vi "GetAlarms.vi"(0 "Valve_2DO_2DI in":refnum<class "Valve_2DO_2DI.lvclass">, 11 "error in (no error)":errorcluster) -> (4 "Valve_2DO_2DI out":refnum<class "Valve_2DO_2DI.lvclass">, 6 "Alarm":bool, 8 "Warning":bool, 15 "error out":errorcluster)   [LabVIEW 2019, in "Valve_2DO_2DI.lvclass"]
uses:
  Valve_2DO_2DI.lvclass
  Valve_2DO_2DI.lvclass/Valve_2DO_2DI.ctl
  DA_class/DA.lvclass
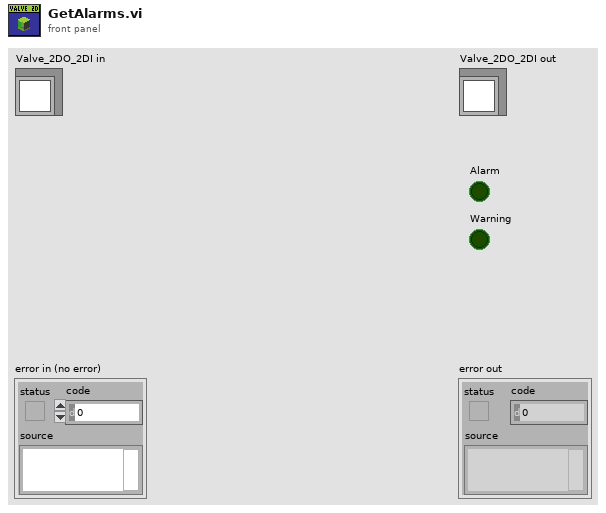
[diagram p1: front panel]
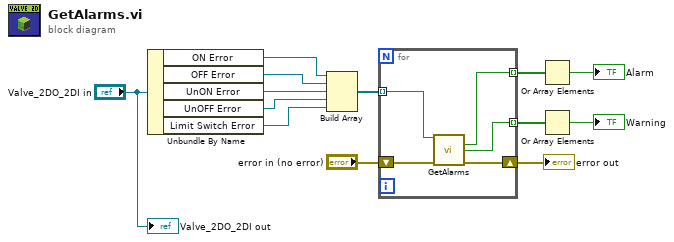
[diagram p0: block diagram]
diagram:
  n1 = Unbundle By Name("Valve_2DO_2DI in") -> ("ON Error"=w12:refnum<class "DA.lvclass">, "OFF Error"=w11:refnum<class "DA.lvclass">, "UnON Error"=w10:refnum<class "DA.lvclass">, "UnOFF Error"=w9:refnum<class "DA.lvclass">, "Limit Switch Error"=w8:refnum<class "DA.lvclass">)
  n2 = Build Array(w12, w11, w10, w9, w8) -> (w7:refnum<class "DA.lvclass">[])
  n3 = for {
    tunnel: w7 -> [w18] mode=indexing
    tunnel: [w17] -> w4 mode=indexing
    tunnel: [w16] -> w3 mode=indexing
    shift-right: [w15] -> w5
    shift-left: "error in (no error)" -> [w14]
    n4 = call-dynamic "GetAlarms.vi"("DA in"=w18, "error in (no error)"=w14) -> ("Alarm"=w17:bool, "Warning"=w16:bool, "error out"=w15:errorcluster)  [unwired: 10 in, 1 out]
  }
  "error out" <- w5
  n5 = Or Array Elements(Boolean array=w4) -> (logical OR=→"Alarm":bool)
  n6 = Or Array Elements(Boolean array=w3) -> (logical OR=→"Warning":bool)
  "Valve_2DO_2DI out" <- "Valve_2DO_2DI in"
